vi "BS the tug main A.vi"() -> ()   [LabVIEW 2012]
uses:
  <vilib>/userdefined/High Color/IMAQdx.ctl
  <vilib>/vision/driver/NI_Vision_Acquisition_Software.lvlib
  <vilib>/vision/NI_Vision_Development_Module.lvlib
panel:
  out "Scaled image":T1(plugin-control)
  out "Running?":bool
  out "All found?":bool
  in  "Data sent":string
  out "error out":errorcluster
  out "Image":T1(plugin-control)
  in  "stop":bool
  in  "Image Type":T2 items=["Grayscale (U8)", "Grayscale (I16)", "Grayscale (SGL)", "Complex (CSG)", "RGB (U32)", "HSL (U32)", "RGB (U64)", "Grayscale (U16)"]
  in  "Session In":T3="cam0"
  # "This VI receives an image from the camera above the pool and modifies the image to be 1032 x 1032 it then:\n1. Locates (4) tugs with greek letter symbols\n2. Locates (4) buoys with circle symbols\n3. Records the time the image is taken\n4. Creates a single string of that data and transmits the string using UDP to port 61557\n\nTO OPERATE START THE ROUTINE!"
  # "The Point Grey camera settings should be:\nAuto Exposure      Auto\nBrightness             Relative     200\nGain                       Auto\nFrame Rate           Absolute   20\nShutter                  Auto\n\nThese values are programmed into this VI\n\nThe overhead lights should be OFF"
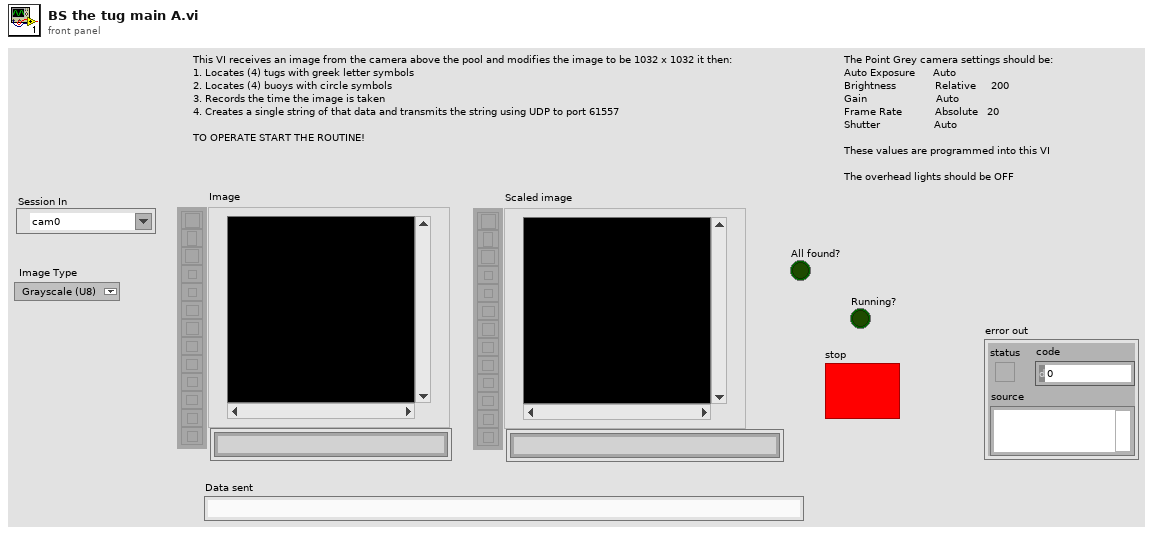
[diagram p1: front panel]
types:
  T1 = typedef "IMAQ Image.ctl" = refnum<image>
  T2 = typedef "Image Type" = u32
  T3 = typedef "IMAQdx.ctl" = refnum<k21>
  T4 = cluster{"Greek Letter":string, i16, i16, i16, bool}[]
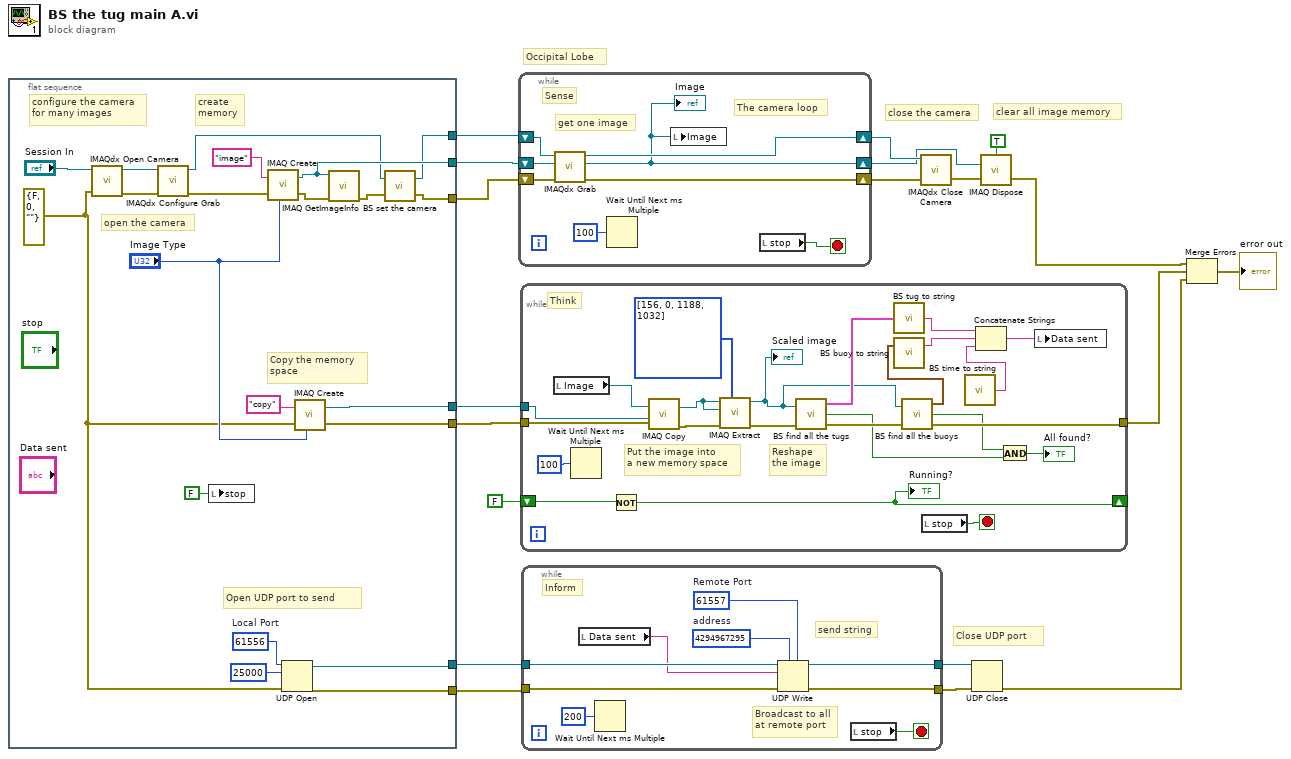
[diagram p0: block diagram]
diagram:
  # "Occipital Lobe"
  # "Close UDP port"
  # "clear all image memory"
  # "close the camera"
  n1 = flat-sequence {
    tunnel: [w23] -> w12
    tunnel: [w21] -> w13
    tunnel: [w34] -> w14
    tunnel: [w31] -> w10
    tunnel: [w30] -> w11
    tunnel: [w27] -> w4
    tunnel: [w26] -> w3
    frame #0 {
      w29 = u16 61556  # Local Port
      w25 = errorcluster {"status"=FALSE, "code"=0, "source"=""} ("error in")
      # "Open UDP port to send"
      # "Copy the memory\nspace"
      # "create\nmemory"
      # "configure the camera\nfor many images"
      # "open the camera"
      n2 = call <vilib>:"IMAQdx Open Camera.vi"("error in"=w25, "Session In"="Session In") -> ("error out"=w37:errorcluster, "Session Out"=w38:T3)  [unwired: 1 in, 7 out]
      n3 = call <vilib>:"IMAQdx Configure Grab.vi"("error in"=w37, "Session In"=w38) -> ("error out"=w39:errorcluster, "Session Out"=w22:T3)  [unwired: 8 out]
      n4 = local write "stop"(FALSE ("stop")) -> ()
      n5 = call "IMAQ Create"("Image Name"="image", "Image Type"="Image Type", "error in (no error)"=w39) -> ("New Image"=w34:T1, "error out"=w40:errorcluster)  [unwired: 1 in, 1 out]
      n6 = UDP Open(8:w25, 9:25000 ("timeout ms (25000)"), 11:w29) -> (port=w26:refnum<k16>, 0:w27:errorcluster)  [unwired: 3 out]
      n7 = call "IMAQ Create"("Image Name"="copy", "Image Type"="Image Type", "error in (no error)"=w25) -> ("New Image"=w30:T1, "error out"=w31:errorcluster)  [unwired: 2 in]
      n8 = call "IMAQ GetImageInfo"("error in (no error)"=w40, "Image"=w34) -> ("error out"=w24:errorcluster)  [unwired: 2 in, 7 out]
      n9 = call "BS set the camera.vi"("error in"=w24, "IMAQdx Session input"=w22) -> ("error out"=w23:errorcluster, "IMAQdx Session output"=w21:T3)
    }
  }
  n10 = while {
    shift-right: [w45] -> w19
    shift-left: w13 -> [w48]
    shift-right: [w41] -> w16
    shift-left: w14 -> [w47]
    shift-right: [w44] -> w18
    shift-left: w12 -> [w46]
    stop <- w42 stop-if-true
    # "Sense"
    # "The camera loop"
    # "get one image"
    n11 = call <vilib>:"IMAQdx Grab.vi"("error in"=w46, "Image In"=w47, "Session In"=w48) -> ("error out"=w44:errorcluster, "Image Out"=w41:T1, "Session Out"=w45:T3)  [unwired: 5 in, 1 out]
    "Image" <- w41
    n12 = Wait Until Next ms Multiple(millisecond multiple=u32 100) -> ()  [unwired: 1 out]
    n13 = local write "Image"(w41) -> ()
    n14 = local read "stop"() -> (w42:bool)
  }
  n15 = while {
    tunnel: w11 -> [w67]
    tunnel: w10 -> [w68]
    tunnel: [w57] -> w8
    shift-right: [w60] -> _
    shift-left: FALSE -> [w61]
    stop <- w63 stop-if-true
    # "Think"
    # "Reshape\nthe image"
    # "Put the image into \na new memory space"
    n16 = local read "Image"() -> (w66:T1)
    n17 = Wait Until Next ms Multiple(millisecond multiple=u32 100) -> ()  [unwired: 1 out]
    n18 = Not(x=w61) -> (.not. x?=w60:bool)
    "Running?" <- w60
    n19 = call "IMAQ Copy"("error in (no error)"=w68, "Image Dst"=w67, "Image Src"=w66) -> ("error out"=w70:errorcluster, "Image Dst Out"=w71:T1)  [unwired: 3 in]
    n20 = call "IMAQ Extract"("Optional Rectangle"=i32[] [156, 0, 1188, 1032], "error in (no error)"=w70, "Image Dst"=w71, "Image Src"=w71) -> ("error out"=w65:errorcluster, "Image Dst Out"=w58:T1)  [unwired: 6 in]
    "Scaled image" <- w58
    n21 = call "BS find all the tugs.vi"("Image Src"=w58, "error in"=w65) -> ("Tug location array"=w64:T4, "All found?"=w53:bool, "error out"=w59:errorcluster)
    n22 = call "BS tug to string.vi"("Tug location array"=w64) -> ("tug location string"=w52:string)
    n23 = call "BS find all the buoys.vi"("Image Src"=w58, "error in"=w59) -> ("Buoy Array"=w55:cluster{i16, i16}[], "Buoys found?"=w54:bool, "error out"=w57:errorcluster)
    n24 = call "BS buoy to string.vi"("Buoy Array"=w55) -> ("Buoy location string"=w51:string)  [unwired: 1 in, 1 out]
    n25 = local read "stop"() -> (w63:bool)
    n26 = call "BS time to string.vi"() -> ("time string"=w50:string)  [unwired: 1 in]
    n27 = Concatenate Strings(w52, w51, w50) -> (w49:string)
    n28 = And(x=w54, y=w53) -> (x .and. y?=→"All found?":bool)
    n29 = local write "Data sent"(w49) -> ()
  }
  n30 = while {
    tunnel: w3 -> [w80]
    tunnel: w4 -> [w79]
    tunnel: [w78] -> w6
    tunnel: [w77] -> w5
    stop <- w73 stop-if-true
    w76 = u16 61557  # Remote Port
    w75 = u32 4294967295  # address
    # "Inform"
    # "send string"
    # "Broadcast to all\nat remote port"
    n31 = local read "Data sent"() -> (w74:string)
    n32 = Wait Until Next ms Multiple(millisecond multiple=u32 200) -> ()  [unwired: 1 out]
    n33 = UDP Write(address=w75, port or service name=w76, connection ID=w80, data in=w74, 8:w79) -> (error out=w78:errorcluster, 3:w77:refnum<k16>)  [unwired: 1 out]
    n34 = local read "stop"() -> (w73:bool)
  }
  n35 = call <vilib>:"IMAQdx Close Camera.vi"("error in"=w18, "Session In"=w19) -> ("error out"=w17:errorcluster)  [unwired: 9 out]
  n36 = UDP Close(connection ID=w5, 8:w6) -> (error out=w2:errorcluster)  [unwired: 1 out]
  n37 = call "IMAQ Dispose"("All Images? (No)"=TRUE, "Image"=w16, "error in (no error)"=w17) -> ("error out"=w9:errorcluster)  [unwired: 3 out]
  n38 = Merge Errors(w9, w8, w2) -> (→"error out":errorcluster)
